vi "SetText.vi"(8 "error in (no error)":errorcluster, 10 "Text":string, 11 "Text in":refnum<class "Text.lvclass">) -> (0 "error out":errorcluster, 3 "Text out":refnum<class "Text.lvclass">)   [LabVIEW 2021, in "Picture2D.lvlib" / "Text.lvclass"]
uses:
  Text.lvclass
  Text.lvclass/Text.ctl
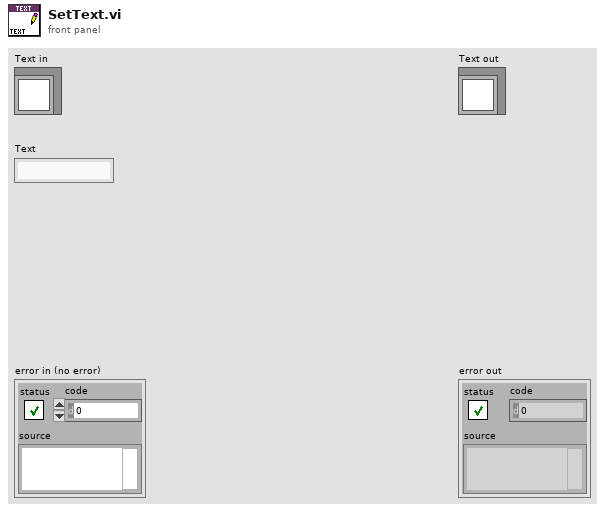
[diagram p1: front panel]
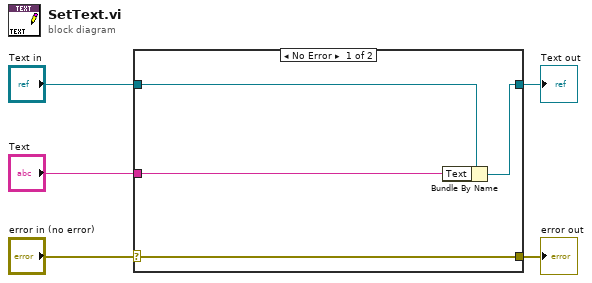
[diagram p0: block diagram]
diagram:
  n1 = case shown="No Error" "error in (no error)" {
    selector: "error in (no error)" -> [w9 w10]
    tunnel: [w9 w10] -> w4
    tunnel: [w7 w11] -> w2
    tunnel: "Text in" -> [w8 w11]
    tunnel: "Text" -> [w6 _]
    frame No Error {
      n2 = Bundle By Name(cluster=w8, "Text"=w6) -> (w7:refnum<class "Text.lvclass">)
    }
    frame Error {
    }
  }
  "error out" <- w4
  "Text out" <- w2
